vi "Control.vi"(7 "Disabled":bool, 8 "Robot Mode":T1, 9 "SensorInputData":T9, 10 "HMI to Control":T4={"RightDriveValue"=0.0, "LeftDriveValue"=0.0, "Arm Manual "=0.0, "Stacker Manual "=0.0, "Claw Manual "=0.0, "ClawSlightOpenNumber"=0, "Intake Value "=0.0, "Arm States"=enum."4 Tote", "Claw States"=enum."Claw Manual ", "Intake Man. or Sense"=enum."Sensing", "Stacker in Manual?"=FALSE, "Drop Stack? "=FALSE, "Tusk Up Request"=FALSE, "Tusk Down Request"=FALSE, "Inver. Wheels  In Request"=FALSE, "Inverse. Wheels Out Request "=FALSE, "Get Out of Manual Control"=FALSE, "Exit Score State"=FALSE, "DriveStraight Help?"=FALSE, "Stacker Shut Off No."=0, "Stacker Need Off?"=FALSE, "Collecting?"=FALSE, "Go to Hover"=FALSE, "Stack Clamp Lock "=FALSE, "Stack Clamp Unlock "=FALSE, "Claw Intake Value "=0.0, "Stack Clamp Lock No. "=0, "Steal Can (ruin their day?)"=FALSE, "Retract (have mercy?)"=FALSE, "Can Grab No. "=0, "Wench Value to Control "=0.0}, 11 "ActuatorInputs":T8) -> (0 "Stacker to Dashboard Out":T2={"# of Totes Out"=0, "Stacker State to Index"=enum."Hold", "Stacker Off?"=FALSE, "Stack Clamp Locked?"=FALSE}, 1 "SensorInputDataOut":T9, 2 "HMI to Control Out":T4={"RightDriveValue"=0.0, "LeftDriveValue"=0.0, "Arm Manual "=0.0, "Stacker Manual "=0.0, "Claw Manual "=0.0, "ClawSlightOpenNumber"=0, "Intake Value "=0.0, "Arm States"=enum."4 Tote", "Claw States"=enum."Claw Manual ", "Intake Man. or Sense"=enum."Sensing", "Stacker in Manual?"=FALSE, "Drop Stack? "=FALSE, "Tusk Up Request"=FALSE, "Tusk Down Request"=FALSE, "Inver. Wheels  In Request"=FALSE, "Inverse. Wheels Out Request "=FALSE, "Get Out of Manual Control"=FALSE, "Exit Score State"=FALSE, "DriveStraight Help?"=FALSE, "Stacker Shut Off No."=0, "Stacker Need Off?"=FALSE, "Collecting?"=FALSE, "Go to Hover"=FALSE, "Stack Clamp Lock "=FALSE, "Stack Clamp Unlock "=FALSE, "Claw Intake Value "=0.0, "Stack Clamp Lock No. "=0, "Steal Can (ruin their day?)"=FALSE, "Retract (have mercy?)"=FALSE, "Can Grab No. "=0, "Wench Value to Control "=0.0}, 3 "ActuatorInputsOut":T8)   [LabVIEW 2014]
uses:
  Typedefs/SensorInputData.ctl
  Typedefs/ActuatorInputs.ctl
  Typedefs/HMI_to_Control.ctl
  Typedefs/Arm States.ctl
  Typedefs/ClawStates.ctl
  Typedefs/IntakeWheelSenseOrManual.ctl
  Typedefs/StackerToDashboardData.ctl
  Typedefs/StackerStates.ctl
  <vilib>/Rock Robotics/WPI/DriverStation/WPI_DriverStationRobotMode2.ctl
panel:
  in  "Stacker to Dashboard":T2={"# of Totes Out"=0, "Stacker State to Index"=enum."Hold", "Stacker Off?"=FALSE, "Stack Clamp Locked?"=FALSE}
  # "s"
  # "s"
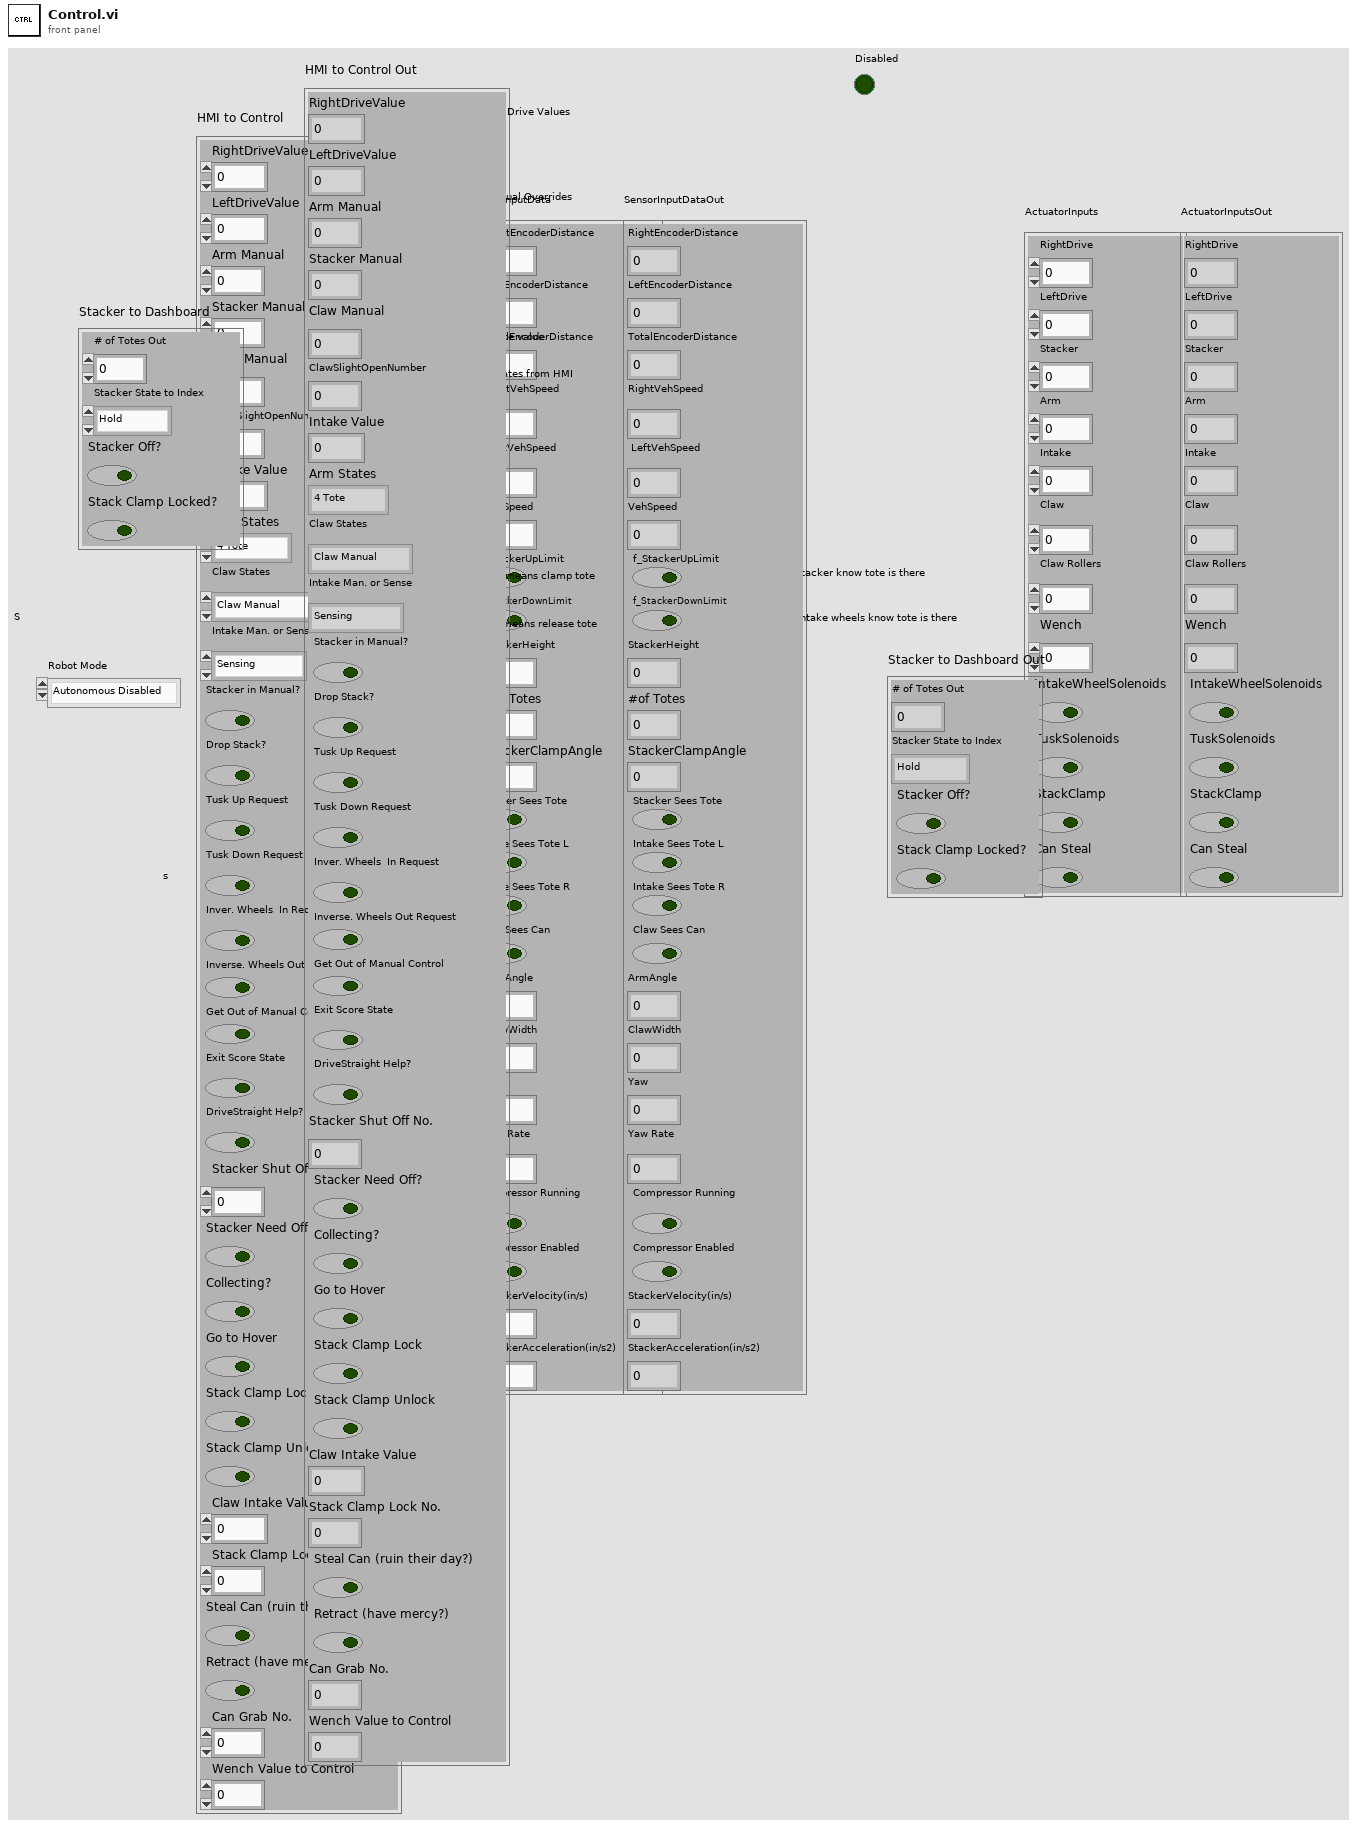
[diagram p1: front panel]
types:
  T1 = typedef "WPI_DriverStationRobotMode2.ctl" = enum16{"Autonomous Disabled", "Autonomous Enabled", "Teleop Disabled", "Teleop Enabled", "Disconnected", "Finish", "Test Disabled", "Test Enabled", "Emergency Stopped"}
  T2 = typedef "StackerToDashboardData.ctl" = cluster{"# of Totes Out":i32, "Stacker State to Index":T3, "Stacker Off?":bool, "Stack Clamp Locked?":bool}
  T3 = typedef "StackerStates.ctl" = enum16{"Manual ", "Hold", "Hold5", "Hold6", "GetTote", "DropStack", "Hover", "Hover5", "Wait for Up", "DecideHold", "DownTimerPeriod", "Prep Intake for Drop", "Check Arm before 5", "Make Arm ready for 5", "Check Arm before 6", "Make Arm ready for 6", "Delay for 5", "Delay for 6"}
  T4 = typedef "HMI_to_Control.ctl" = cluster{"RightDriveValue":dbl, "LeftDriveValue":dbl, "Arm Manual ":dbl, "Stacker Manual ":dbl, "Claw Manual ":dbl, "ClawSlightOpenNumber":i8, "Intake Value ":sgl, "Arm States":T5, "Claw States":T6, "Intake Man. or Sense":T7, "Stacker in Manual?":bool, "Drop Stack? ":bool, "Tusk Up Request":bool, "Tusk Down Request":bool, "Inver. Wheels  In Request":bool, "Inverse. Wheels Out Request ":bool, "Get Out of Manual Control":bool, "Exit Score State":bool, "DriveStraight Help?":bool, "Stacker Shut Off No.":i8, "Stacker Need Off?":bool, "Collecting?":bool, "Go to Hover":bool, "Stack Clamp Lock ":bool, "Stack Clamp Unlock ":bool, "Claw Intake Value ":sgl, "Stack Clamp Lock No. ":i8, "Steal Can (ruin their day?)":bool, "Retract (have mercy?)":bool, "Can Grab No. ":i8, "Wench Value to Control ":dbl}
  T5 = typedef "Arm States.ctl" = enum16{"Arm Manual ", "Ground", "Step", "1 Tote", "2 Tote", "3 Tote", "4 Tote", "5 Tote", "6 Tote", "Flip Can Arm", "Grab Can in auto", "Nudge"}
  T6 = typedef "ClawStates.ctl" = enum16{"Claw Manual ", "Claw Open", "Claw Closed", "Claw Slight Open", "Flip Can"}
  T7 = typedef "IntakeWheelSenseOrManual.ctl" = enum16{"Sensing", "Manual "}
  T8 = typedef "ActuatorInputs.ctl" = cluster{"RightDrive":dbl, "LeftDrive":dbl, "Stacker":dbl, "Arm":dbl, "Intake":sgl, "Claw":dbl, "Claw Rollers":i8, "Wench":dbl, "IntakeWheelSolenoids":bool, "TuskSolenoids":bool, "StackClamp":bool, "Can Steal":bool}
  T9 = typedef "SensorInputData.ctl" = cluster{"RightEncoderDistance":dbl, "LeftEncoderDistance":dbl, "TotalEncoderDistance":dbl, "RightVehSpeed":dbl, "LeftVehSpeed":dbl, "VehSpeed":dbl, "f_StackerUpLimit":bool, "f_StackerDownLimit":bool, "StackerHeight":dbl, "#of Totes":u8, "StackerClampAngle":dbl, "Stacker Sees Tote":bool, "Intake Sees Tote L":bool, "Intake Sees Tote R":bool, "Claw Sees Can":bool, "ArmAngle":dbl, "ClawWidth":dbl, "Yaw":dbl, "Yaw Rate":dbl, "Compressor Running":bool, "Compressor Enabled":bool, "StackerVelocity(in/s)":dbl, "StackerAcceleration(in/s2)":dbl}
  T10 = typedef "IntakeWheelStates.ctl" = enum16{"Intake Wheels Open", "Intake Wheels Closed", "Decide off of Input", "Delay before Close", "Operator Request"}
  T11 = typedef "TuskStates.ctl" = enum16{"Down", "Up"}
  T12 = typedef "Can Grabber.ctl" = enum16{"Do not steal ", "Steal "}
  T13 = typedef "StackClampStates.ctl" = enum16{"Unlock", "Lock"}
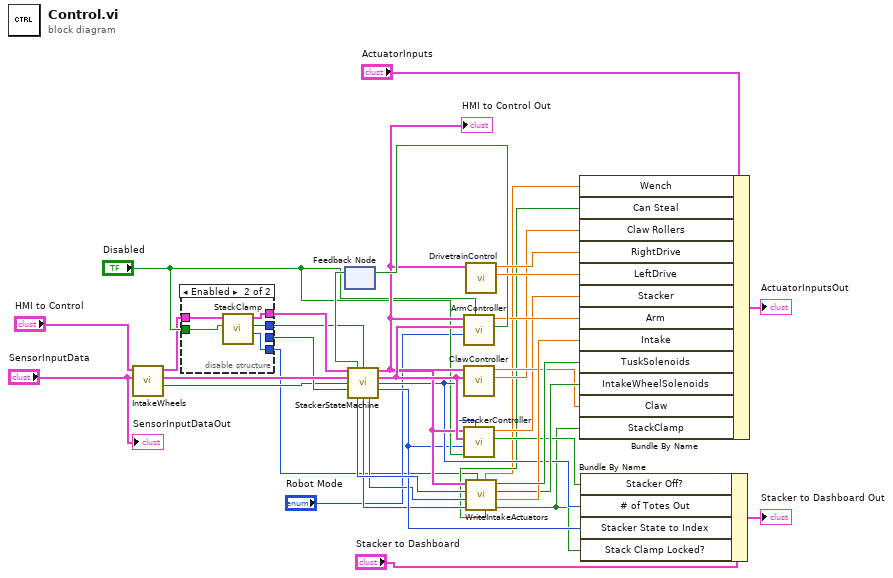
[diagram p0: block diagram]
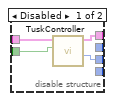
[diagram p2: hidden frame]
diagram:
  n1 = call "IntakeWheels.vi"("SensorInputData"="SensorInputData", "HMI to Control"="HMI to Control") -> ("Intake Wheel State Out"=w9:T10, "SensorInputData Out"=w36:T9, "HMI to Control  Out"=w11:T4)  [unwired: 6 in, 1 out]
  n2 = disable-structure shown="Enabled" {
    disable-tunnel: [w40 _] -> w30
    disable-tunnel: [w39 w45] -> w28
    disable-tunnel: "Disabled" -> [w38 w44]
    disable-tunnel: w11 -> [w41 w46]
    disable-tunnel: [_ w43] -> w10
    disable-tunnel: [_ w42] -> w2
    frame Disabled {
      n3 = call "TuskController.vi"("Disabled"=w38, "HMI to Control"=w41) -> ("Tusk State Out"=w40:T11, "HMI to Control  Out"=w39:T4)  [unwired: 7 in, 1 out]
    }
    frame Enabled {
      n4 = call "StackClamp.vi"("Disabled"=w44, "HMI to Control"=w46) -> ("CanGrabStateOut"=w42:T12, "StackClampStateOut"=w43:T13, "HMI to Control  Out"=w45:T4)  [unwired: 7 in]
    }
  }
  n5 = feedback #1() -> (w26:bool)  [unwired: 1 in]
  n6 = call "StackerStateMachine.vi"("HMI to Control"=w28, "Arm Arrived"=w26, "StackClampState"=w10, "SensorInputData"=w36, "Intake Wheel State"=w9, "Tusk State"=w30) -> ("HMI to Control  Out"=w20:T4, "SensorInputData out"=w22:T9, "# of Totes Out"=w16:i32, "Stacker State to Index"=w13:T3, "Tusk State to Actuate"=w29:T11, "StackClampState to Actuate"=w7:T13, "Intake Wheel State to Actuate"=w8:T10)  [unwired: 2 in, 1 out]
  "HMI to Control Out" <- w20
  n7 = call "ArmController.vi"("Disabled"="Disabled", "RobotMode"="Robot Mode", "SensorInputData"=w22, "HMI to Control"=w20) -> ("Device has arrived"=w27:bool, "Final Arm Output"=w19:dbl)  [unwired: 6 in]
  n8 = feedback-in #1(w27) -> ()
  n9 = call "ClawController.vi"("SensorInputData"=w22, "HMI to Control"=w20) -> ("Claw Intake Value"=w6:dbl, "Claw Final Output"=w21:dbl)  [unwired: 8 in]
  n10 = call "StackerController.vi"("HMI to Control"=w20, "SensorInputData"=w22, "StackerStates"=w13, "Disabled?"="Disabled", "Number of Totes"=w16) -> ("Final Stacker Output"=w12:dbl, "Stacker Off?"=w18:bool)  [unwired: 4 in]
  n11 = call "DrivetrainControl.vi"("HMI to Control"=w20) -> ("LeftDriveFinalOutput"=w34:dbl, "RightDriveFinalOutput"=w35:dbl)  [unwired: 9 in]
  n12 = call "WriteIntakeActuators.vi"("CanGrabStates"=w2, "StackClampStates"=w7, "Intake Wheel States"=w8, "Tusk State"=w29, "HMI to Control"=w20) -> ("Stack Clamp Output"=w5:bool, "Intake Value"=w31:sgl, "Intake Wheel Solenoid Output"=w23:bool, "Tusk Solenoid Output"=w32:bool, "Can Grab Output"=w3:bool, "Wench Value to Control"=w1:dbl)  [unwired: 1 in]
  n13 = Bundle By Name(cluster="ActuatorInputs", "Wench"=w1, "Can Steal"=w3, "Claw Rollers"=w6, "RightDrive"=w35, "LeftDrive"=w34, "Stacker"=w12, "Arm"=w19, "Intake"=w31, "TuskSolenoids"=w32, "IntakeWheelSolenoids"=w23, "Claw"=w21, "StackClamp"=w5) -> (→"ActuatorInputsOut":T8)
  n14 = Bundle By Name(cluster="Stacker to Dashboard", "Stacker Off?"=w18, "# of Totes Out"=w16, "Stacker State to Index"=w13, "Stack Clamp Locked?"=w5) -> (→"Stacker to Dashboard Out":T2)
  "SensorInputDataOut" <- "SensorInputData"
